vi "SVL Exp Avg Sound Level (N ch).vi"(6 "restart averaging (F)":bool, 8 "error in (no error)":errorcluster, 9 "time constant [ms]":dbl=125.0 format="%.2f", 10 "exponential mode":enum16{"Slow", "Fast", "Impulse", "Custom"}(ring)=enum."Fast", 11 "scaled signals [EU]":waveform(dbl)[](array[waveform])) -> (0 "error out":errorcluster, 1 "actual time constant [ms]":dbl=nan format="%.2f", 2 "unit labels":string[](array[string]), 3 "exp avg sound levels [dB EU]":waveform(dbl)[](array[waveform]), 4 "maximum sound levels [dB EU]":dbl[](array[numeric]) format="%.2f")   [LabVIEW 2017, in "SoundVib_SoundLevel.lvlib"]
doc: "Computes the exponential averaged sound level of <B>scaled signal [EU]</B>. <B>scaled signal [EU]</B> should have a zero DC component. Wire data to the <B>scaled signal [EU]</B> input to determine the polymorphic instance to use or manually select the instance."
uses:
  <vilib>/addons/Sound and Vibration/svt_Level/SoundVib_SoundLevel.lvlib
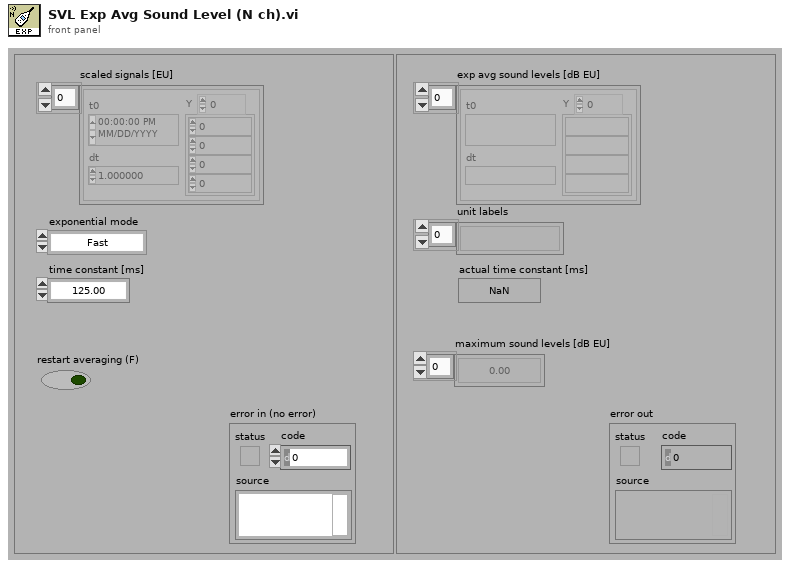
[diagram p1: front panel]
types:
  T1 = enum16{"RMS", "Running RMS", "Exp avg  ", "Dec exp avg ", "Peak", "Crest"}
  T2 = enum16{"Reset filter", "Restart averaging", "Continue processing"}
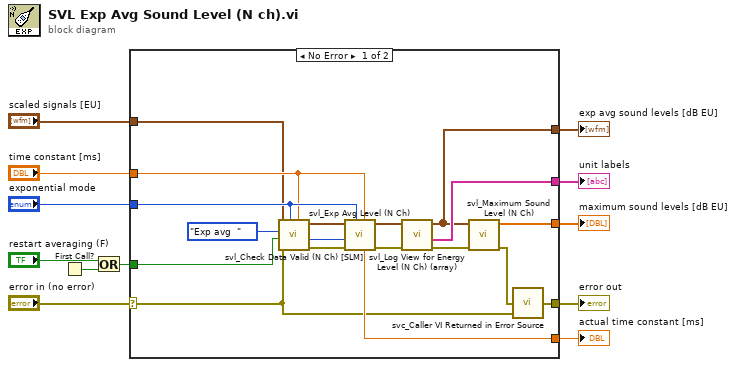
[diagram p0: block diagram]
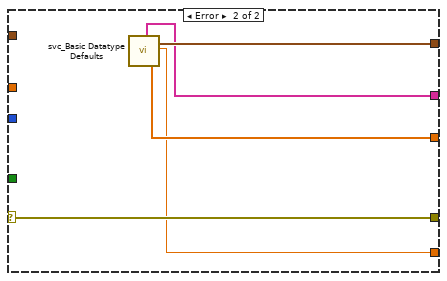
[diagram p2: hidden frame]
diagram:
  n1 = First Call?() -> (First Call?: T/F=w7:bool)
  n2 = Or(x="restart averaging (F)", y=w7) -> (x .or. y?=w6:bool)
  n3 = case shown="No Error" "error in (no error)" {
    selector: "error in (no error)" -> [w13 w35]
    tunnel: [w21 w35] -> w12
    tunnel: [w27 w33] -> w11
    tunnel: [w14 w34] -> w10
    tunnel: "scaled signals [EU]" -> [w16 _]
    tunnel: w6 -> [w26 _]
    tunnel: "exponential mode" -> [w24 _]
    tunnel: "time constant [ms]" -> [w23 _]
    tunnel: [w22 w31] -> w3
    tunnel: [w18 w32] -> w1
    frame No Error {
      n4 = call <vilib>:"svl_Check Data Valid (N Ch) [SLM].vi"("time constant [ms]"=w23, "exponential mode"=w24, "error in (no error)"=w13, "restart averaging (F)"=w26, "level analysis"=T1."Exp avg  " ("Level Analysis"), "scaled signals [EU]"=w16) -> ("error out"=w30:errorcluster, "processing state"=w25:T2, "dup scaled signals [EU]"=w15:waveform(dbl)[])  [unwired: 3 in]
      n5 = call <vilib>:"svl_Exp Avg Level (N Ch).vi"("timeConstant"=w23, "exponential mode"=w24, "error in (no error)"=w30, "processing state"=w25, "scaled signals"=w15) -> ("error out"=w29:errorcluster, "exp avg signals"=w28:waveform(dbl)[], "actual time constant [ms]"=w22:dbl)  [unwired: 3 in, 1 out]
      n6 = call <vilib>:"svl_Log View for Energy Level (N Ch) (array).vi"("error in (no error)"=w29, "scaled signals"=w28) -> ("error out"=w20:errorcluster, "unit labels"=w27:string[], "scaled signals"=w14:waveform(dbl)[])  [unwired: 7 in]
      n7 = call <vilib>:"svl_Maximum Sound Level (N Ch).vi"("error in (no error)"=w20, "scaled signals"=w14) -> ("error out"=w19:errorcluster, "maximum sound levels [dB EU]"=w18:dbl[])  [unwired: 8 in]
      n8 = call <vilib>:"svc_Caller VI Returned in Error Source.vi"("warning input to caller"=w13, "error in (no error)"=w19) -> ("error out"=w21:errorcluster)  [unwired: 3 in]
    }
    frame Error {
      n9 = call <vilib>:"svc_Basic Datatype Defaults.vi"() -> ("empty array of strings"=w33:string[], "empty array of DBL"=w32:dbl[], "empty array of waveforms"=w34:waveform(dbl)[], "NaN"=w31:dbl)  [unwired: 7 in, 9 out]
    }
  }
  "exp avg sound levels [dB EU]" <- w10
  "actual time constant [ms]" <- w3
  "unit labels" <- w11
  "error out" <- w12
  "maximum sound levels [dB EU]" <- w1
